vi "Init.vi"(8 "error in (no error)":errorcluster, 11 "uService Template in":refnum<class "New uService Template.lvclass">) -> (0 "error out":errorcluster, 3 "uService Template out":refnum<class "New uService Template.lvclass">)   [LabVIEW 2020, in "New uService Template.lvlib" / "New uService Template.lvclass"]
uses:
  New uService Template.lvclass
  TALOS/TALOS_PPL.lvlibp/Father of all uServices/Father of all uServices/Father of all uServices.lvclass
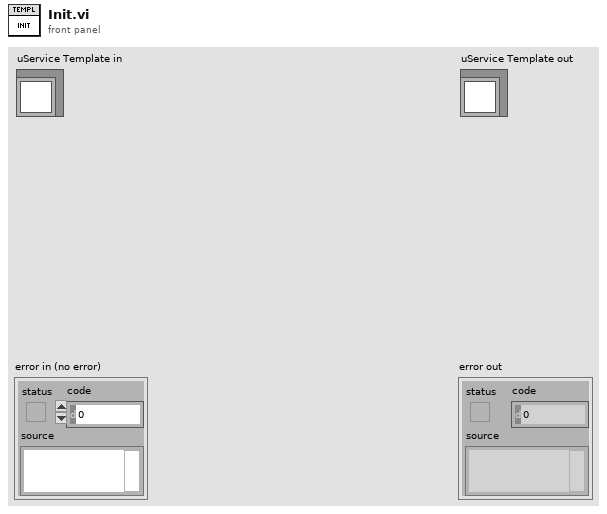
[diagram p1: front panel]
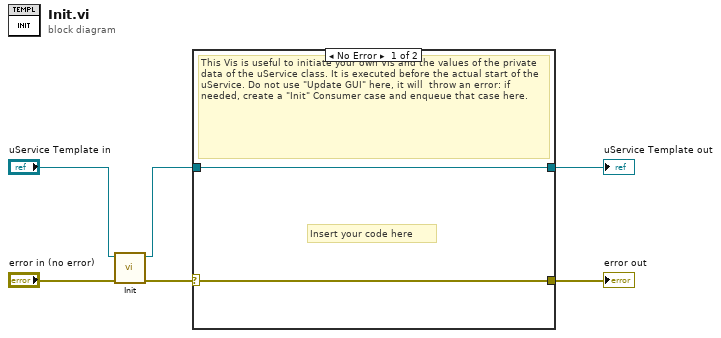
[diagram p0: block diagram]
diagram:
  n1 = call-parent "Init.vi"("error in (no error)"="error in (no error)", "uService Template in"="uService Template in") -> ("error out"=w3:errorcluster, "uService Template out"=w1:refnum<class "New uService Template.lvclass">)  [unwired: 8 in]
  n2 = case shown="No Error" w3 {
    selector: w3 -> [w7 w9]
    tunnel: w1 -> [w8 w10]
    tunnel: [w8 w10] -> w6
    tunnel: [w7 w9] -> w5
    frame No Error {
      # "Insert your code here"
      # "This Vis is useful to initiate your own VIs and the values of the private data of the uService class. It is executed before the actual start of the uService. Do not use \"Update GUI\" here, it will  throw an error: if needed, create a \"Init\" Consumer case and enqueue that case here."
    }
    frame Error {
    }
  }
  "error out" <- w5
  "uService Template out" <- w6
